vi "7-1.vi"() -> ()   [LabVIEW 2019, in "7.lvlib"]
uses:
  7.lvlib
panel:
  out "total fuel":i32
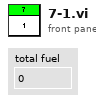
[diagram p1: front panel]
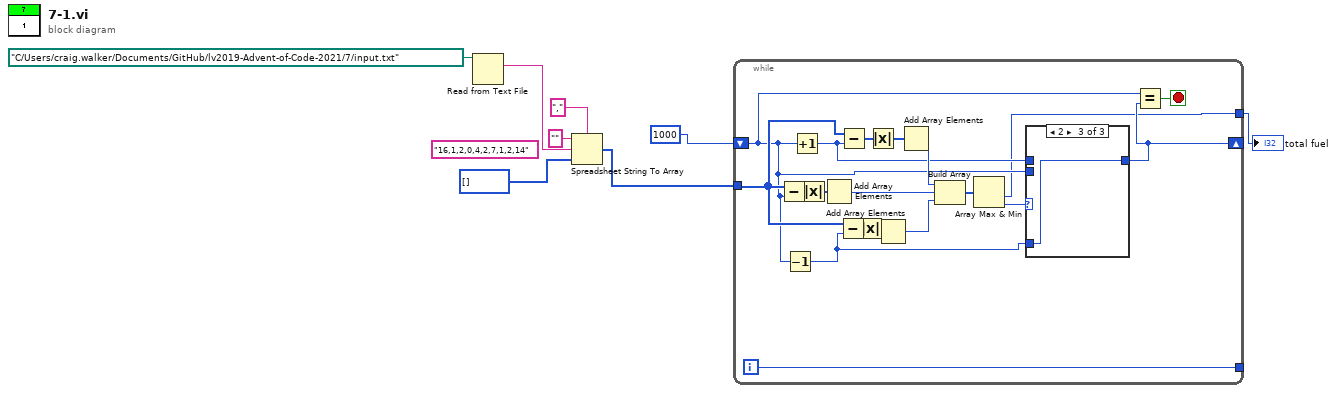
[diagram p0: block diagram]
diagram:
  (unwired) "16,1,2,0,4,2,7,1,2,14"
  n1 = Read from Text File(file (use dialog)=path "C:/Users/craig.walker/Documents/GitHub/lv2019-Advent-of-Code-2021/7/input.txt") -> (text=w4:string)  [unwired: 3 in, 3 out]
  n2 = Spreadsheet String To Array(delimiter (Tab)=",", format string="", spreadsheet string=w4, array type (2D Dbl)=i32[] []) -> (array=w5:i32[])
  n3 = while {
    tunnel: w5 -> [w26]
    shift-right: [w16] -> _
    shift-left: 1000 ("Numeric") -> [w15]
    tunnel: [w10] -> _
    tunnel: [w9] -> w1
    i -> [w10]
    stop <- w14 stop-if-true
    n4 = Subtract(x=w26, y=w15) -> (x-y=w27:i32[])
    n5 = Decrement(x=w15) -> (x-1=w17:i32)
    n6 = Increment(x=w15) -> (x+1=w18:i32)
    n7 = Absolute Value(x=w27) -> (abs(x)=w12:i32[])
    n8 = Add Array Elements(numeric array=w12) -> (sum=w22:i32)
    n9 = Subtract(x=w26, y=w17) -> (x-y=w24:i32[])
    n10 = Subtract(x=w26, y=w18) -> (x-y=w25:i32[])
    n11 = Absolute Value(x=w24) -> (abs(x)=w11:i32[])
    n12 = Absolute Value(x=w25) -> (abs(x)=w13:i32[])
    n13 = Add Array Elements(numeric array=w11) -> (sum=w21:i32)
    n14 = Add Array Elements(numeric array=w13) -> (sum=w23:i32)
    n15 = Build Array(w23, w22, w21) -> (w20:i32[])
    n16 = Array Max & Min(array=w20) -> (min value=w9:i32, min index (indices)=w19:i32)  [unwired: 2 out]
    n17 = case shown="2" w19 {
      tunnel: w18 -> [w28 _ _]
      tunnel: [w28 w29 w30] -> w16
      tunnel: w15 -> [_ w29 _]
      tunnel: w17 -> [_ _ w30]
      frame 0, Default {
      }
      frame 1 {
      }
      frame 2 {
      }
    }
    n18 = Equal?(x=w15, y=w16) -> (x = y?=w14:bool)
  }
  "total fuel" <- w1
